vi "VDUT ON.vi"(1 "error in (no error)":errorcluster, 3 "Device address":i32=4660 format="%x") -> (0 "error out":errorcluster)   [LabVIEW 2011]
doc: "Turns on Vdut power for USB DAQ and USB DIG."
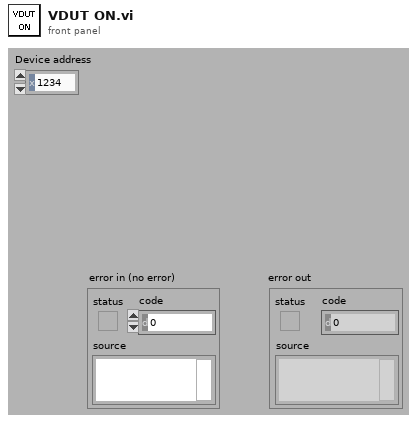
[diagram p1: front panel]
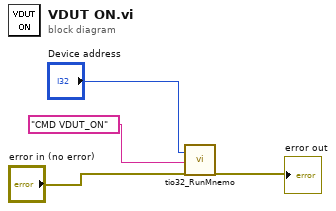
[diagram p0: block diagram]
diagram:
  n1 = call "tio32_RunMnemo.vi"("Device address"="Device address", "command string"="CMD VDUT_ON", "error in (no error)"="error in (no error)") -> ("error out"=→"error out":errorcluster)  [unwired: 6 in, 10 out]
